vi "Pills Inspector.vi"() -> ()   [LabVIEW 2017]
doc: "Printed Circuit Board Inspection\nDetermine whether PCB components are present and in the correct location using pattern matching. Match areas of inspection to a template of valid components. Use shift-invariant matching to inspect an oriented component (diode). Use rotation-invariant matching to inspect an unoriented component (resistor)."
uses:
  IMAQCV/IMAQCV.lvlib
  IMAQCV/LVOpenCV.lvlib
panel:
  in  "Image Delay ms":u32=5000
  out "Image":T1(plugin-control)
  in  "Template Path":path=path "c:/vision/Pills/Template Pill.png"
  out "Number of Pills":i32
  in  "Image File path":path=path "c:/vision/Pills/Blister1.jpg"
  out "Image Log path":path=path "c:/vision/Result.jpg"
  out "error out":errorcluster
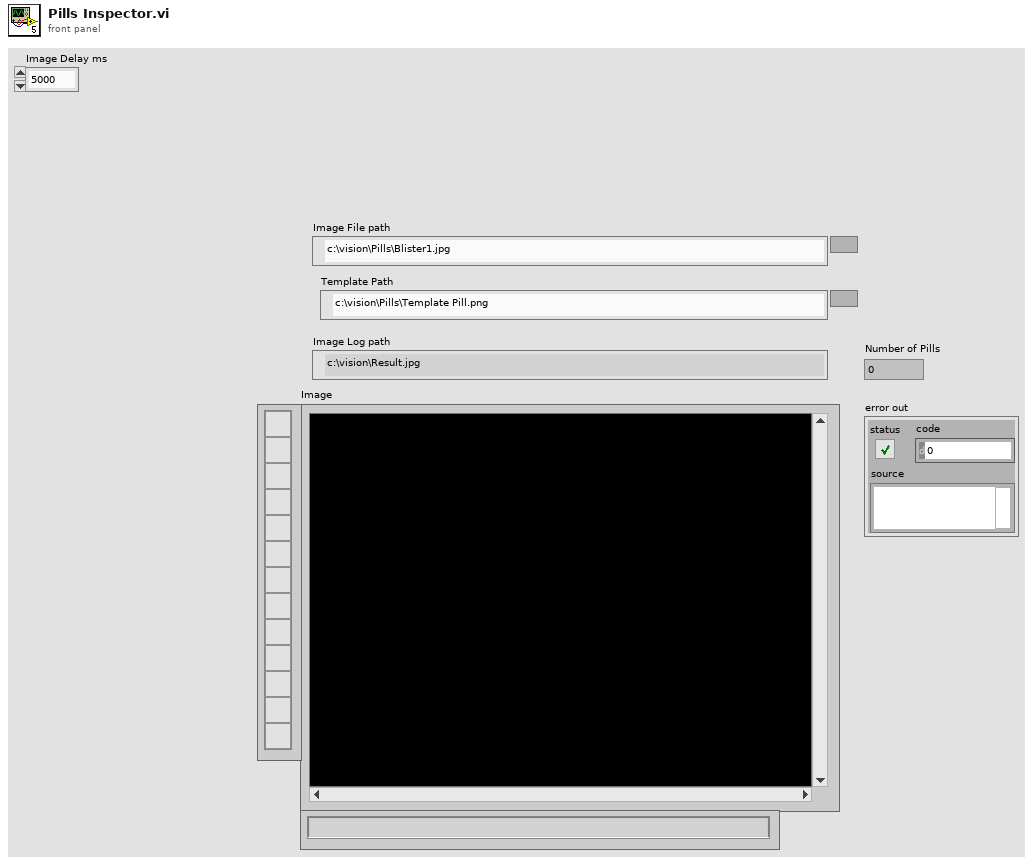
[diagram p1: front panel]
types:
  T1 = typedef "IMAQ Image.ctl" = refnum<image>
  T2 = cluster{"Global Rectangle":i32[], "Contours":cluster{"ID":enum32{"External", "Internal"}, "Type":u32, "Coordinates":i32[]}[]}
  T3 = typedef "Image Type" = u32
  T4 = cluster{"Position":cluster{"x":sgl, "y":sgl}, "Angle":sgl, "Scale":sgl, "Score":sgl, "Bounding Box":cluster{"x":sgl, "y":sgl}[]}[]
  T5 = typedef "IMAQCV.lvlib/IMAQCV Image.ctl" = refnum<vi>
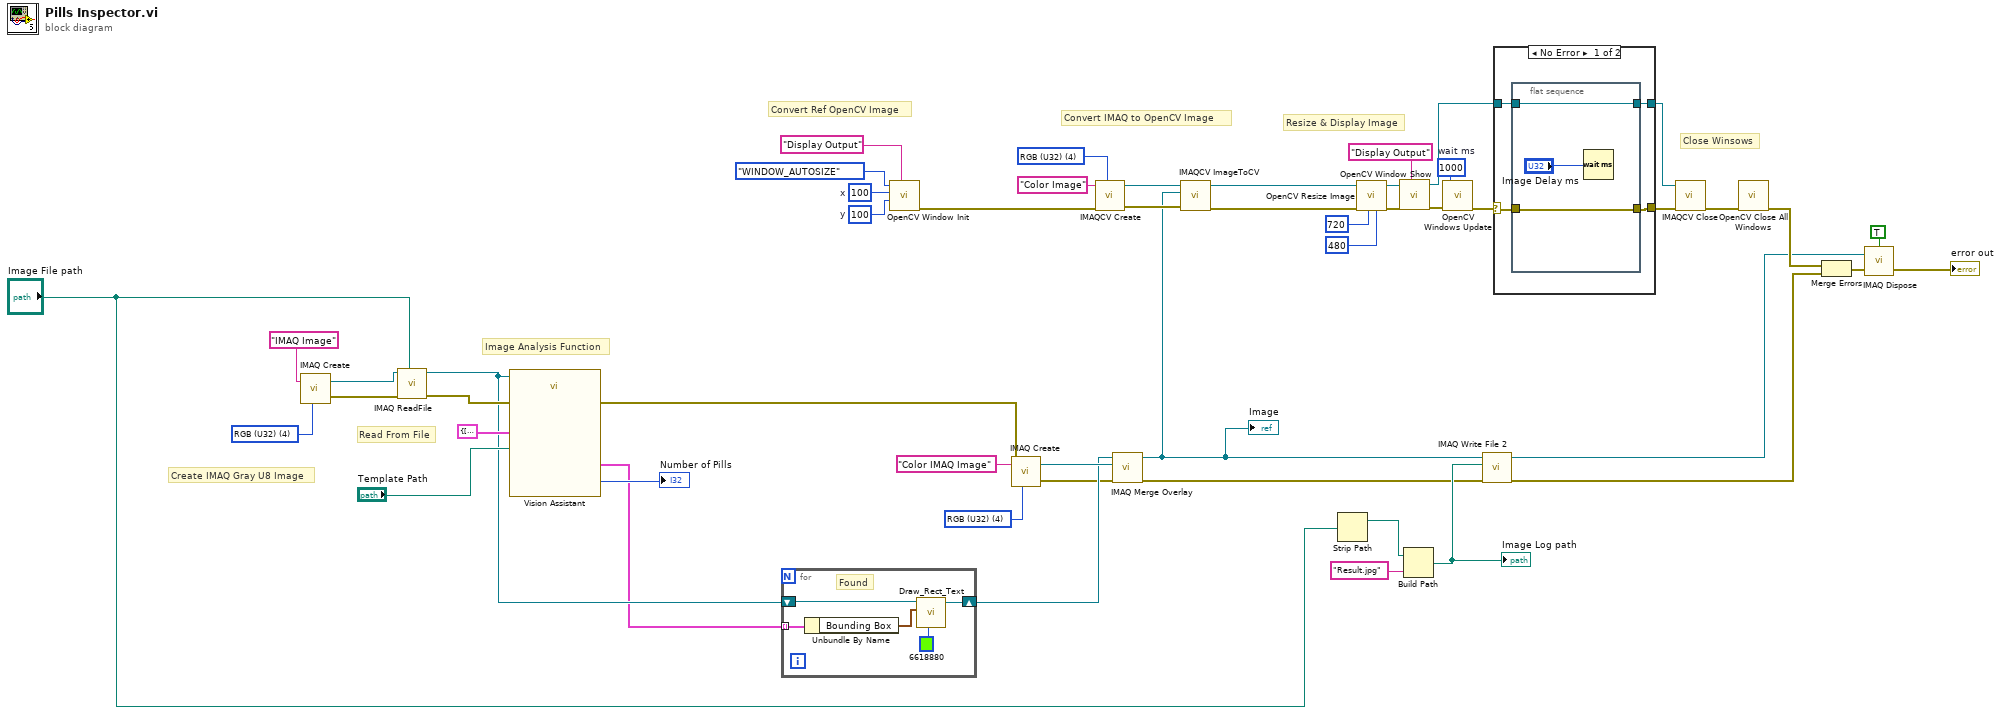
[diagram p0: block diagram]
diagram:
  w21 = 1000  # wait ms
  w28 = u32 100  # y
  w29 = u32 100  # x
  w32 = u32 4 items=["Grayscale (U8)", "Grayscale (I16)", "Grayscale (SGL)", "Complex (CSG)", "RGB (U32)", "HSL (U32)", "RGB (U64)", "Grayscale (U16)"] ("Image Type")
  w2 = T3 4 items=["Grayscale (U8)", "Grayscale (I16)", "Grayscale (SGL)", "Complex (CSG)", "RGB (U32)", "HSL (U32)", "RGB (U64)", "Grayscale (U16)"] ("Image Type")
  w1 = T3 4 items=["Grayscale (U8)", "Grayscale (I16)", "Grayscale (SGL)", "Complex (CSG)", "RGB (U32)", "HSL (U32)", "RGB (U64)", "Grayscale (U16)"] ("Image Type")
  # "Close Winsows"
  # "Resize & Display Image"
  # "Convert Ref OpenCV Image"
  # "Convert IMAQ to OpenCV Image"
  # "Image Analysis Function"
  # "Read From File"
  # "Create IMAQ Gray U8 Image"
  n1 = call "IMAQ Create"("Image Name"="IMAQ Image", "Image Type"=w1) -> ("New Image"=w50:T1, "error out"=w49:errorcluster)  [unwired: 2 in, 1 out]
  n2 = call "IMAQ ReadFile"("File Path"="Image File path", "error in (no error)"=w49, "Image"=w50) -> ("error out"=w41:errorcluster, "Image Out"=w37:T1)  [unwired: 2 in, 5 out]
  n3 = call "Vision Assistant"("Image In"=w37, "ROI Descriptor (Color Location 1)"=T2 {"Global Rectangle"=[0, 0, 319, 239], "Contours"=[{"ID"=enum."External", "Type"=12, "Coordinates"=[0, 0, 319, 239, 0]}]}, "File Path (Color Location 1)"="Template Path", "error in"=w41) -> ("Matches (Color Location 1)"=w35:T4, "Number of Matches (Color Location 1)"=→"Number of Pills":i32, "error out"=w3:errorcluster)  [unwired: 20 in, 1 out]
  n4 = for {
    shift-right: [w54] -> w36
    shift-left: w37 -> [w56]
    tunnel: w35 -> [w53] mode=indexing
    # "Found"
    n5 = Unbundle By Name(w53) -> ("Bounding Box"=w52:cluster{"x":sgl, "y":sgl}[])
    n6 = call "Draw_Rect_Text.vi"("Color"=u32 6618880, "Bounding Box"=w52, "Image"=w56) -> ("Image 2"=w54:T1)  [unwired: 7 in, 1 out]
  }
  n7 = call "OpenCV Window Init.vi"("window name"="Display Output", "y"=w28, "x"=w29, "mode"=enum8{"WINDOW_AUTOSIZE", "WINDOW_FULLSCREEN"}."WINDOW_AUTOSIZE") -> ("error out"=w12:errorcluster)  [unwired: 7 in]
  n8 = call "IMAQ Create"("Image Name"="Color IMAQ Image", "Image Type"=w2, "error in (no error)"=w3) -> ("New Image"=w47:T1, "error out"=w4:errorcluster)  [unwired: 1 in, 1 out]
  n9 = call "IMAQCV Create.vi"("Image Type"=w32, "error in (no error)"=w12, "Image Name"="Color Image") -> ("error out"=w15:errorcluster, "Image Out"=w33:T5)  [unwired: 7 in]
  n10 = call "IMAQ Merge Overlay"("error in (no error)"=w4, "Image Dst"=w47, "Image Src"=w36) -> ("error out"=w42:errorcluster, "Image Dst Out"=w5:T1)  [unwired: 7 in]
  "Image" <- w5
  n11 = call "IMAQCV ImageToCV.vi"("error in (no error)"=w15, "Variant In"=w5, "CV in"=w33) -> ("error out"=w11:errorcluster, "CV out"=w20:T5)  [unwired: 7 in]
  n12 = Strip Path(path="Image File path") -> (stripped path=w45:path)  [unwired: 1 out]
  n13 = call "OpenCV Resize Image.vi"("height"=u32 480, "width"=u32 720, "error in (no error)"=w11, "image in"=w20) -> ("error out"=w24:errorcluster, "image out"=w25:T5)  [unwired: 6 in]
  n14 = call "OpenCV Window Show.vi"("window name"="Display Output", "error in (no error)"=w24, "image in"=w25) -> ("error out"=w26:errorcluster, "image out"=w18:T5)  [unwired: 7 in]
  n15 = Build Path(base path=w45, name or relative path="Result.jpg") -> (appended path=w43:path)
  "Image Log path" <- w43
  n16 = call "OpenCV Windows Update.vi"("error in (no error)"=w26, "wait ms"=w21) -> ("error out"=w14:errorcluster)  [unwired: 8 in, 1 out]
  n17 = call-poly "IMAQ Write File 2"("error in (no error)"=w42, "File Path"=w43, "Image"=w5) -> ("error out"=w7:errorcluster, "Image Out (duplicate)"=w8:T1)  [unwired: 7 in]
  n18 = case shown="No Error" w14 {
    selector: w14 -> [w57 w65]
    tunnel: [w60 w65] -> w19
    tunnel: w18 -> [w59 w64]
    tunnel: [w58 w64] -> w17
    frame No Error {
      n19 = flat-sequence {
        tunnel: [w63] -> w60
        tunnel: w57 -> [w63]
        tunnel: [w62] -> w58
        tunnel: w59 -> [w62]
        frame #0 {
          n20 = Wait (ms)(milliseconds to wait="Image Delay ms") -> ()  [unwired: 1 out]
        }
      }
    }
    frame Error {
    }
  }
  n21 = call "IMAQCV Close.vi"("error in (no error)"=w19, "Image"=w17) -> ("error out"=w16:errorcluster)  [unwired: 9 in]
  n22 = call "OpenCV Close All Windows.vi"("error in (no error)"=w16) -> ("error out"=w9:errorcluster)  [unwired: 10 in]
  n23 = Merge Errors(w9, w7) -> (w10:errorcluster)
  n24 = call "IMAQ Dispose"("All Images? (No)"=TRUE, "Image"=w8, "error in (no error)"=w10) -> ("error out"=→"error out":errorcluster)  [unwired: 3 in]
